vi "test_Series Simluated DO PWM Tacho Fans.vi"(8 "Error In":errorcluster) -> (0 "Error Out":errorcluster)   [LabVIEW 2023]
uses:
  Series/Series Base/Series Base.lvclass
  <vilib>/ActorFramework/Actor/Actor.lvclass
  Series/Series Actor/Series Actor/Series Actor.lvclass
  8bd81235-fcfd-4522-8496-46042de7d728.vi
  DIO/DIO DAQmx Simulated CFGs/DO DAQmx PWM Fixed Freq CFG/DO DAQmx Fixed Freq PWM CFG.lvclass
  DIO/Virtual DIO/Virt PWM Fixed Freq Generator/Virt DAQmx Fixed Freq PWM Generator.lvclass
  Sample Series/Sample PWM Fans/Sample PWM Fans/Sample PWM Fans.lvclass
panel:
  in  "Stop Button":bool
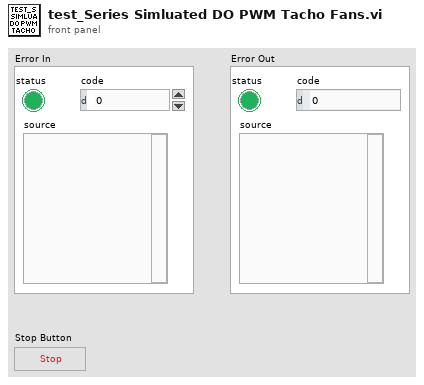
[diagram p1: front panel]
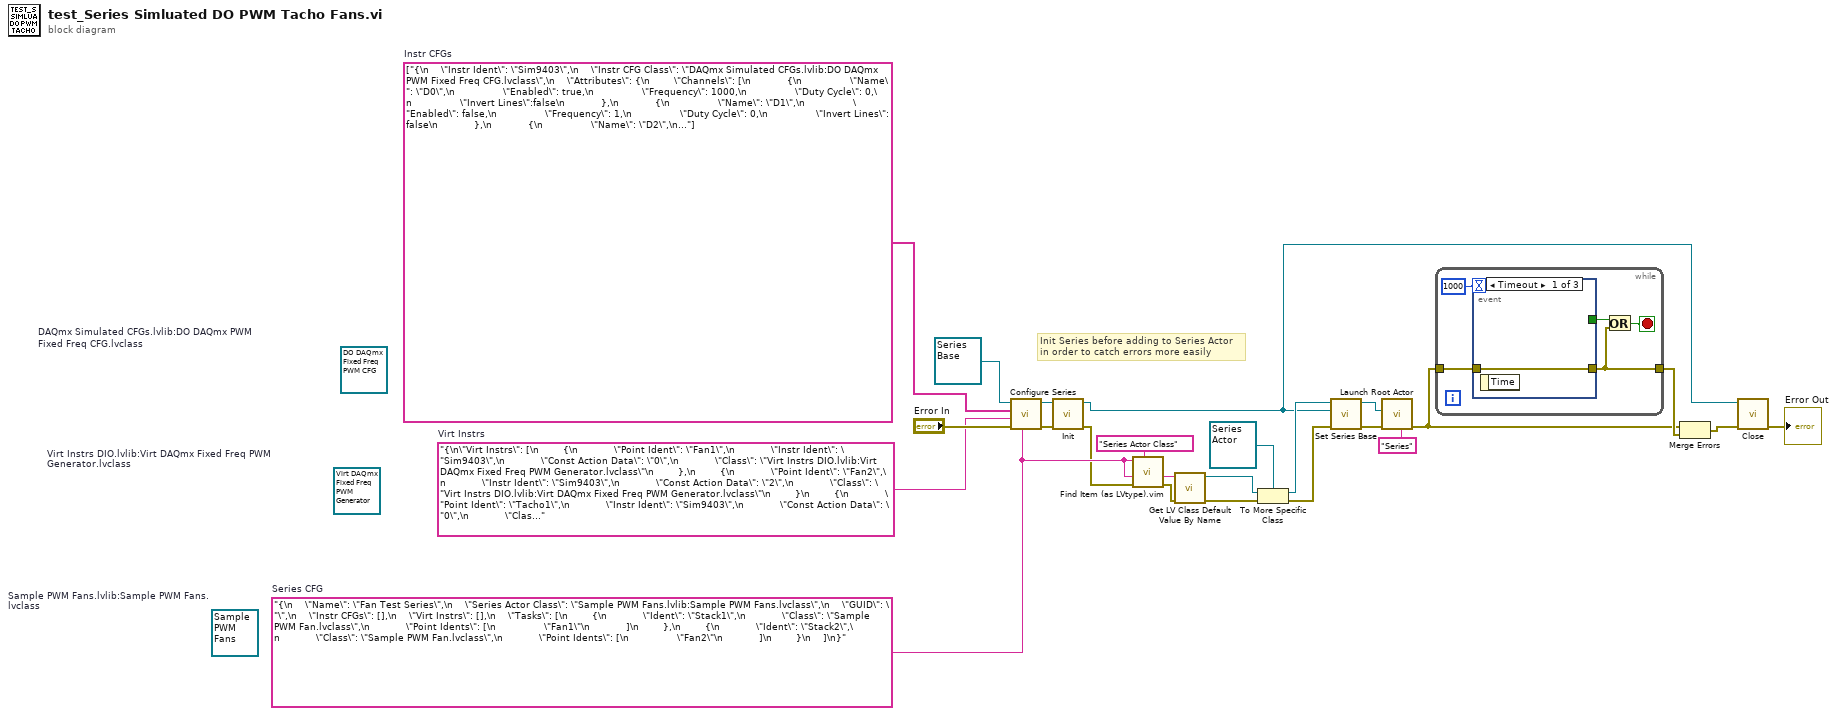
[diagram p0: block diagram]
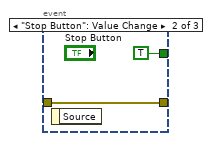
[diagram p2: hidden frame]
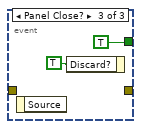
[diagram p3: hidden frame]
diagram:
  (unwired) refnum<class "Sample PWM Fans.lvclass"> refnum  # Sample PWM Fans.lvlib:Sample PWM Fans.lvclass
  (unwired) refnum<class "Virt DAQmx Fixed Freq PWM Generator.lvclass"> refnum  # Virt Instrs DIO.lvlib:Virt DAQmx Fixed Freq PWM Generator.lvclass
  (unwired) refnum<class "DO DAQmx Fixed Freq PWM CFG.lvclass"> refnum  # DAQmx Simulated CFGs.lvlib:DO DAQmx PWM Fixed Freq CFG.lvclass
  w18 = "{\n\"Virt Instrs\": [\n        {\n            \"Point Ident\": \"Fan1\",\n            \"Instr Ident\": \"Sim9403\",\n            \"Const Action Data\": \"0\",\n            \"Class\": \"Virt Instrs DIO.lvlib:Virt DAQmx Fixed Freq PWM Generator.lvclass\"\n        },\n        {\n            \"Point Ident\": \"Fan2\",\n            \"Instr Ident\": \"Sim9403\",\n            \"Const Action Data\": \"2\",\n            \"Class\": \"Virt Instrs DIO.lvlib:Virt DAQmx Fixed Freq PWM Generator.lvclass\"\n        }\n        {\n            \"Point Ident\": \"Tacho1\",\n            \"Instr Ident\": \"Sim9403\",\n            \"Const Action Data\": \"0\",\n            \"Class\": \"Virt Instrs DIO.lvlib:Virt DAQmx Fixed Freq PWM Generator.lvclass\"\n        },\n        {\n            \"Point Ident\": \"Tacho2\",\n            \"Instr Ident\": \"Sim9403\",\n            \"Const Action Data\": \"0\",\n            \"Class\": \"Virt Instrs DIO.lvlib:Virt DAQmx Fixed Freq PWM Generator.lvclass\"\n        },\n    ]\n}"  # Virt Instrs
  w17 = string[] ["{\n    \"Instr Ident\": \"Sim9403\",\n    \"Instr CFG Class\": \"DAQmx Simulated CFGs.lvlib:DO DAQmx PWM Fixed Freq CFG.lvclass\",\n    \"Attributes\": {\n        \"Channels\": [\n            {\n                \"Name\": \"D0\",\n                \"Enabled\": true,\n                \"Frequency\": 1000,\n                \"Duty Cycle\": 0,\n                \"Invert Lines\":false\n            },\n            {\n                \"Name\": \"D1\",\n                \"Enabled\": false,\n                \"Frequency\": 1,\n                \"Duty Cycle\": 0,\n                \"Invert Lines\": false\n            },\n            {\n                \"Name\": \"D2\",\n                \"Enabled\": true,\n                \"Frequency\": 600,\n                \"Duty Cycle\": 0,\n                \"Invert Lines\": false\n            }\n        ],\n        \"Timing\": {\n            \"Type\" : \"Sample Clock\"\n            \"Samples per Channel\": 10000,\n            \"Sample Mode\": \"Continuous Samples\",\n            \"Sample Rate\": 100000,\n            \"Sample Clock Source\": \"OnboardClock\",\n            \"Active Edge\": \"Rising\"\n        },\n        \"Trigger\": {\n            \"Trigger Type\": \"No Trigger\"\n        },\n        \"Generation\": {\n            \"Regen Mode\": \"Allow Regeneration\"\n        }\n    }\n}"]  # Instr CFGs
  w12 = "{\n    \"Name\": \"Fan Test Series\",\n    \"Series Actor Class\": \"Sample PWM Fans.lvlib:Sample PWM Fans.lvclass\",\n    \"GUID\": \"\",\n    \"Instr CFGs\": [],\n    \"Virt Instrs\": [],\n    \"Tasks\": [\n        {\n            \"Ident\": \"Stack1\",\n            \"Class\": \"Sample PWM Fan.lvclass\",\n            \"Point Idents\": [\n                \"Fan1\"\n            ]\n        },\n        {\n            \"Ident\": \"Stack2\",\n            \"Class\": \"Sample PWM Fan.lvclass\",\n            \"Point Idents\": [\n                \"Fan2\"\n            ]\n        }\n    ]\n}"  # Series CFG
  # "Init Series before adding to Series Actor\nin order to catch errors more easily"
  n1 = call "Configure Series.vi"("Series CFG"=w12, "error in (no error)"="Error In", "Virt Instrs CFG"=w18, "Instr CFGs"=w17, "HAL GOOP4:Series Base in"=refnum<class "Series Base.lvclass"> refnum ("HAL GOOP4.lvlib:Study Base.lvclass")) -> ("error out"=w22:errorcluster, "HAL GOOP4:Series Base out"=w20:refnum<class "Series Base.lvclass">)  [unwired: 5 in]
  n2 = call-dynamic "Init.vi"("error in"=w22, "HAL GOOP4:Series Base in"=w20) -> ("error out"=w9:errorcluster, "HAL GOOP4:Series Base out"=w4:refnum<class "Series Base.lvclass">)  [unwired: 8 in]
  n3 = call "Find Item (as LVtype).vim"("$Path or Item Name"="Series Actor Class", "error in (no error)"=w9, "Data Type and Default Value"=w12, "JSON"=w12) -> ("error out"=w10:errorcluster, "Data"=w11:string)  [unwired: 4 in, 2 out]
  n4 = call <vilib>:"Get LV Class Default Value By Name.vi"("error in (no error)"=w10, "class name"=w11) -> ("error out"=w15:errorcluster, "object"=w14:refnum<class>)  [unwired: 8 in]
  n5 = To More Specific Class(target class=refnum<class "Series Actor.lvclass"> refnum ("Series Actor.lvlib:Series Actor.lvclass"), reference=w14, error in=w15) -> (specific class reference=w6:refnum<class "Series Actor.lvclass">, error out=w8:errorcluster)
  n6 = call "Set Series Base.vi"("error in (no error)"=w8, "Series Base"=w4, "Series Actor in"=w6) -> ("error out"=w16:errorcluster, "Series Actor out"=w23:refnum<class "Series Actor.lvclass">)  [unwired: 7 in]
  n7 = call <vilib>:"Launch Root Actor.vi"("Debug Alias"="Series", "error in (no error)"=w16, "Actor"=w23) -> ("error out"=w1:errorcluster)  [unwired: 7 in, 1 out]
  n8 = while {
    tunnel: [w26] -> w2
    tunnel: w1 -> [w29]
    stop <- w27 stop-if-true
    n9 = event shown="[0] Timeout" {
      selector: _ -> [_ _ _]
      dyn-events: _ -> [_ _ _]
      timeout: 1000 -> [_ _ _]
      tunnel: [_ TRUE TRUE] -> w28
      tunnel: [w30 w31 _] -> w26
      tunnel: w29 -> [w30 w31 _]
      event Timeout {
        n10 = event-data() -> ()  [unwired: 1 in, 1 out]
      }
      event "Stop Button": Value Change {
        n11 = event-data() -> ()  [unwired: 1 in, 1 out]
      }
      event Panel Close? {
        n12 = event-data() -> ()  [unwired: 1 in, 1 out]
        n13 = event-data("Discard?"=TRUE) -> ()  [unwired: 1 in, 1 out]
      }
    }
    n14 = Or(x=w28, y=w26) -> (x .or. y?=w27:bool)
  }
  n15 = Merge Errors(w1, w2) -> (w3:errorcluster)
  n16 = call-dynamic "Close.vi"("error in"=w3, "Series Base in"=w4) -> ("error out"=→"Error Out":errorcluster)  [unwired: 8 in, 1 out]
